vi "Temperature Limit.vi"() -> ()   [LabVIEW 2017]
doc: "This VI simulates the acquisition of temperature, graphs the temperature, and notifies the user if the temperature is over the limit."
panel:
  in  "Start":bool
  in  "Delta t (ms)":i32(slide)=400 scale=50.0..500.0
  in  "Stop":bool
  in  "High Limit":dbl=28.0 format="%.2f"
  out "Temperature":cluster{"Temperature":dbl, "High Limit":dbl}(graph)={"Temperature"=85.88749999999999, "High Limit"=80.0}
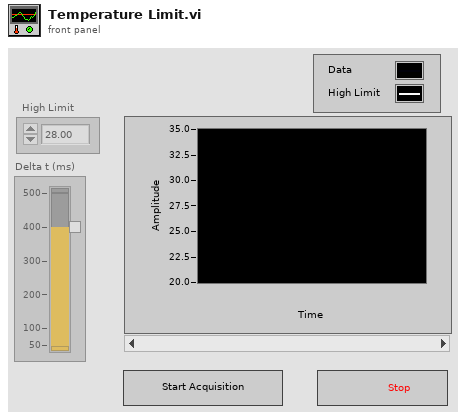
[diagram p1: front panel]
types:
  T1 = enum8{"Enabled", "Disabled", "Disabled and Grayed Out"}
  T2 = cluster{"Temperature Value":dbl, "High Limit":dbl}
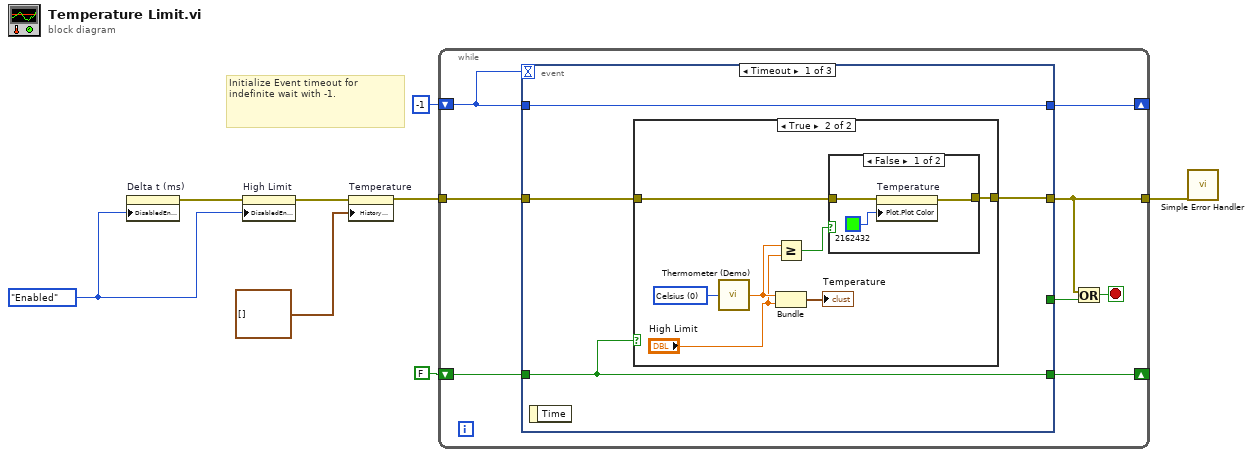
[diagram p0: block diagram]
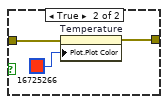
[diagram p3: hidden frame]
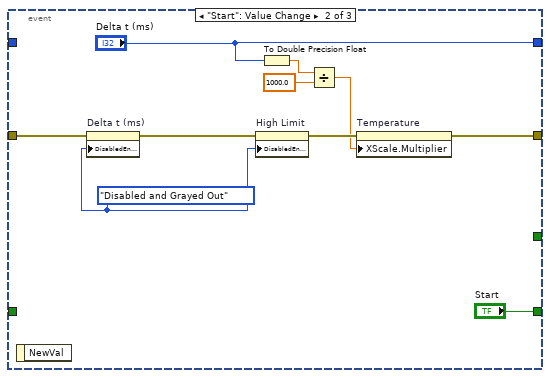
[diagram p4: hidden frame]
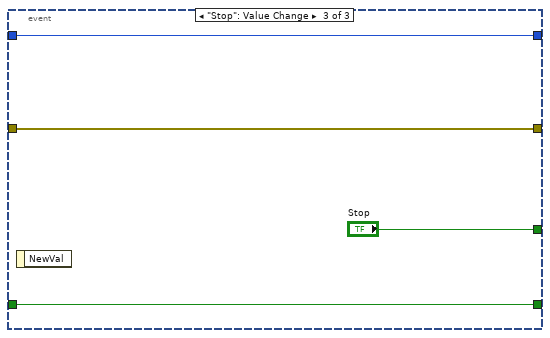
[diagram p5: hidden frame]
diagram:
  w4 = T1."Enabled" ("Disabled")
  # "Initialize Event timeout for indefinite wait with -1."
  n1 = property on="Delta t (ms)" class="Slide (strict)"("DisabledEnum"=w4) -> (error out=w5:errorcluster)  [unwired: 2 in, 1 out]
  n2 = property on="High Limit" class="DigNum (strict)"(error in=w5, "DisabledEnum"=w4) -> (error out=w3:errorcluster)  [unwired: 1 in, 1 out]
  n3 = property on="Temperature" class="WFChart (strict)"(error in=w3, "History Data"=cluster{"Temperature":dbl, "High Limit":dbl}[] []) -> (error out=w2:errorcluster)  [unwired: 1 in, 1 out]
  n4 = while {
    tunnel: w2 -> [w16]
    tunnel: [w14] -> w7
    shift-right: [w12] -> _
    shift-left: FALSE ("Start") -> [w11]
    shift-right: [w10] -> _
    shift-left: -1 ("Delta t (ms)") -> [w9]
    stop <- w15 stop-if-true
    n5 = event shown="[0] Timeout" {
      selector: _ -> [_ _ _]
      dyn-events: _ -> [_ _ _]
      timeout: w9 -> [_ _ _]
      tunnel: [_ _ "Stop"] -> w13
      tunnel: w16 -> [w18 w43 w47]
      tunnel: [w17 w40 w47] -> w14
      tunnel: [w19 "Start" w46] -> w12
      tunnel: w11 -> [w19 _ w46]
      tunnel: [w20 "Delta t (ms)" w45] -> w10
      tunnel: w9 -> [w20 _ w45]
      event Timeout {
        n6 = event-data() -> ()  [unwired: 1 in, 1 out]
        n7 = case shown="True" w19 {
          tunnel: w18 -> [w21 w26]
          tunnel: [w21 w25] -> w17
          frame False {
          }
          frame True {
            w27 = u16 0 items=["Celsius", "Fahrenheit"] ("Units (0: Celsius)")
            n8 = call "Thermometer (Demo).vi"("Units (0: Celsius)"=w27) -> ("Temperature Value"=w24:dbl)
            n9 = Greater Or Equal?(x=w24, y="High Limit") -> (x >= y?=w22:bool)
            n10 = Bundle("Temperature Value"=w24, "High Limit"="High Limit") -> (→"Temperature":T2)  [unwired: 1 in]
            n11 = case shown="False" w22 {
              tunnel: w26 -> [w31 w34]
              tunnel: [w30 w33] -> w25
              frame False {
                n12 = property on="Temperature" class="WFChart (strict)"(error in=w31, "Plot.Plot Color"=u32 2162432) -> (error out=w30:errorcluster)  [unwired: 1 in, 1 out]
              }
              frame True {
                n13 = property on="Temperature" class="WFChart (strict)"(error in=w34, "Plot.Plot Color"=u32 16725266) -> (error out=w33:errorcluster)  [unwired: 1 in, 1 out]
              }
            }
          }
        }
      }
      event "Start": Value Change {
        w35 = T1."Disabled and Grayed Out" ("Disabled")
        n14 = event-data() -> ()  [unwired: 1 in, 1 out]
        n15 = property on="Delta t (ms)" class="Slide (strict)"(error in=w43, "DisabledEnum"=w35) -> (error out=w42:errorcluster)  [unwired: 1 in, 1 out]
        n16 = property on="High Limit" class="DigNum (strict)"(error in=w42, "DisabledEnum"=w35) -> (error out=w41:errorcluster)  [unwired: 1 in, 1 out]
        n17 = To Double Precision Float(number="Delta t (ms)") -> (double precision float=w38:dbl)
        n18 = Divide(x=w38, y=1000.0) -> (x/y=w36:dbl)
        n19 = property on="Temperature" class="WFChart (strict)"(error in=w41, "XScale.Multiplier"=w36) -> (error out=w40:errorcluster)  [unwired: 1 in, 1 out]
      }
      event "Stop": Value Change {
        n20 = event-data() -> ()  [unwired: 1 in, 1 out]
      }
    }
    n21 = Or(x=w14, y=w13) -> (x .or. y?=w15:bool)
  }
  n22 = call <vilib>:"Simple Error Handler.vi"("error in (no error)"=w7) -> ()  [unwired: 4 in, 5 out]
